vi "RDS Child Receive Message.vi"(8 "error in (no error)":errorcluster, 10 "RDS Message":refnum<class "RDS Message.lvclass">, 11 "Battery Instrument in":refnum<class "Battery Instrument.lvclass">) -> (0 "error out":errorcluster, 3 "Battery Instrument out":refnum<class "Battery Instrument.lvclass">)   [LabVIEW 2015, in "Battery Instrument.lvlib" / "Battery Instrument.lvclass"]
uses:
  Battery Instrument.lvclass
  Libraries/RDS Framework/RDS Message Class/RDS Message.lvclass
  Libraries/RDS Framework/RDS Message Class/RDS Message.lvclass/RDS Message.ctl
  Libraries/RDS Serial Handler/RDS Serial Frame.lvclass/RDS Serial Frame.ctl
  <vilib>/ActorFramework/Actor/Actor.lvclass/Actor.ctl
  <vilib>/ActorFramework/Message Enqueuer/Message Enqueuer.lvclass/Message Enqueuer.ctl
  <vilib>/ActorFramework/Message Enqueuer/Enqueue.vi
  <vilib>/ActorFramework/Message Priority Queue/Priority Enqueue.vi
  Libraries/RDS Serial Handler/RDS Serial Frame.lvclass
  <vilib>/ActorFramework/Stop Msg/Stop Msg.lvclass
  Actors/RDS Serial Instrument Actor/RDS Serial Instrument Actor.lvclass
  <vilib>/ActorFramework/Actor/Actor.lvclass
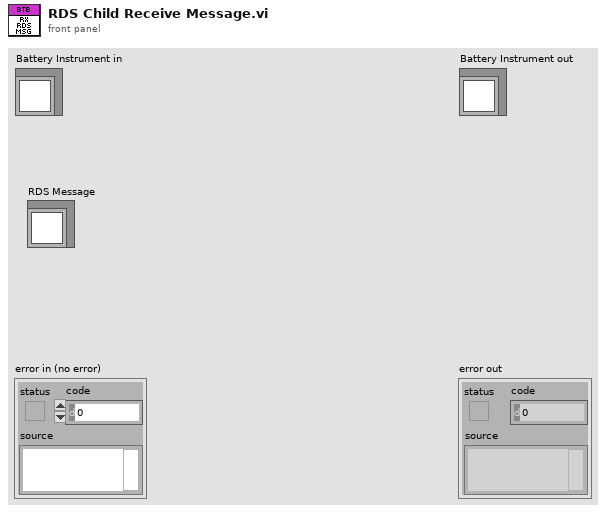
[diagram p1: front panel]
types:
  T1 = typedef "RDS Child Messages.lvlib/RDS Message ID.ctl" = enum16{"RDS Hello World", "String Message", "AIP_Status", "AIP_Command", "GPS_Data", "MCB_Command", "MCB_Status", "Compass_Data", "Depth_Data", "Battery_Data", "Contoller_State", "Set_Mag_Dev", "BTB_Shutdown", "State_Sample_Request", "State_Sample", "PID_Gains_Set", "Helm_Limiter_Set", "Helm_Heading_Command", "Helm_Steering_Command", "Helm_Status", "Controller_Message", "AIP_Set_Min_Depth", "Mission_Controller_State", "Mission_Upload", "Mission_Set_Op_and_Run", "Mission_Settings_Set"}
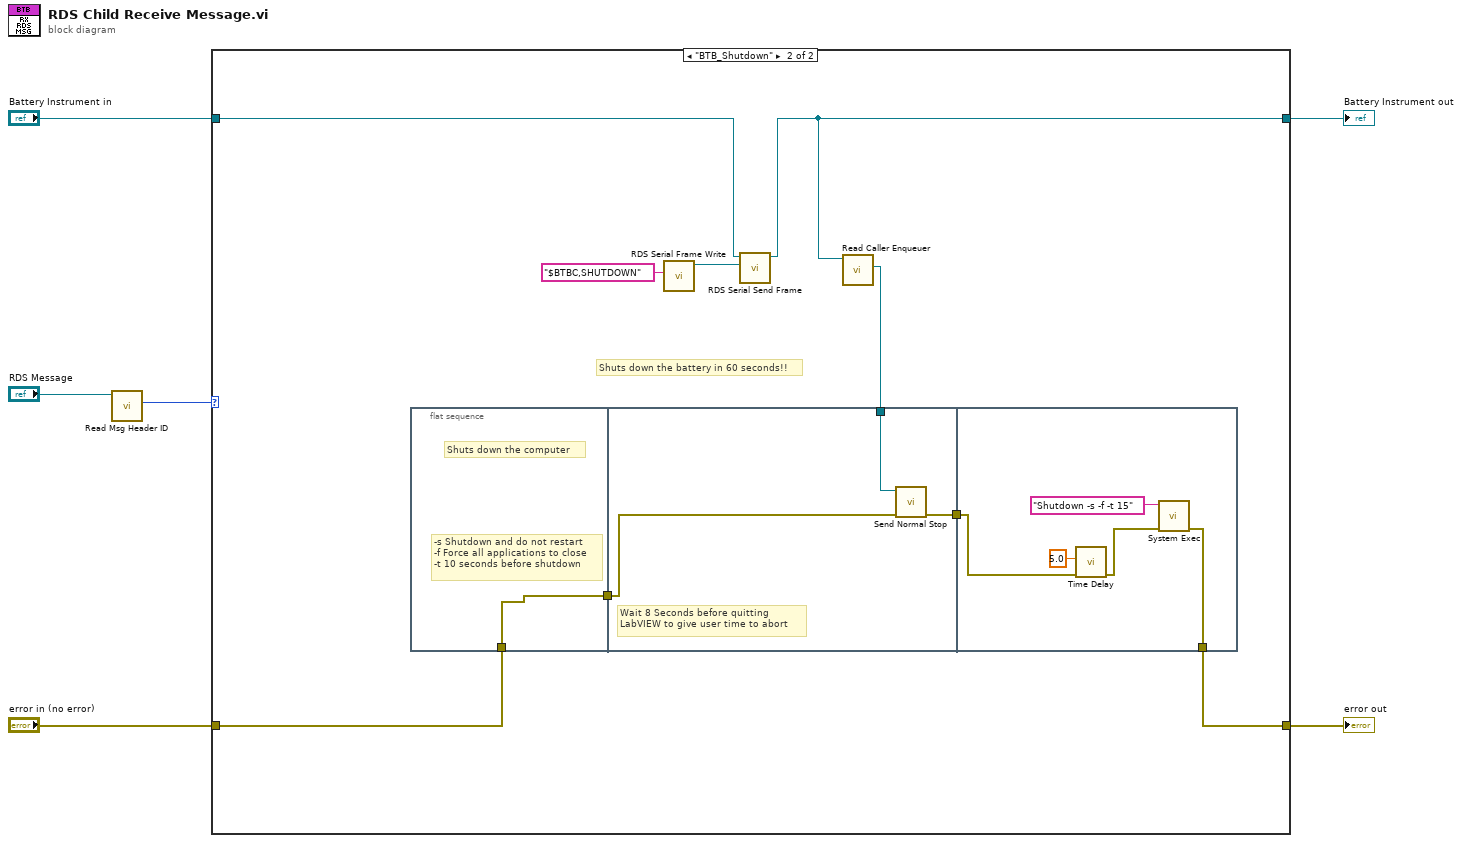
[diagram p0: block diagram]
diagram:
  n1 = call "Read Msg Header ID.vi"("RDS Message in"="RDS Message") -> ("Msg ID"=w3:T1)  [unwired: 6 in, 4 out]
  n2 = case shown="\"BTB_Shutdown\"" w3 {
    tunnel: [w7 w12] -> w6
    tunnel: "Battery Instrument in" -> [w7 w15]
    tunnel: [w8 w9] -> w2
    tunnel: "error in (no error)" -> [w8 w13]
    frame "RDS Hello World", Default {
    }
    frame "BTB_Shutdown" {
      # "Shuts down the battery in 60 seconds!!"
      n3 = flat-sequence {
        tunnel: [w18] -> w14
        tunnel: w13 -> [w18]
        tunnel: w14 -> [w19]
        tunnel: w11 -> [w21]
        tunnel: [w20] -> w10
        tunnel: w10 -> [w24]
        tunnel: [w22] -> w9
        frame #0 {
          # "-s Shutdown and do not restart\n-f Force all applications to close\n-t 10 seconds before shutdown"
          # "Shuts down the computer"
        }
        frame #1 {
          # "Wait 8 Seconds before quitting\nLabVIEW to give user time to abort"
          n4 = call <vilib>:"Send Normal Stop.vi"("error in (no error)"=w19, "Message Enqueuer"=w21) -> ("error out"=w20:errorcluster)  [unwired: 9 in]
        }
        frame #2 {
          n5 = call "Time Delay"("error in (no error)"=w24, "Delay Time (s)"=5.0) -> ("error out"=w23:errorcluster)  [unwired: 9 in]
          n6 = call <vilib>:"System Exec.vi"("error in (no error)"=w23, "command line"="Shutdown -s -f -t 15") -> ("error out"=w22:errorcluster)  [unwired: 6 in, 3 out]
        }
      }
      n7 = call "RDS Serial Frame Write.vi"("Serial String"="$BTBC,SHUTDOWN") -> ("RDS Serial Frame out"=w16:refnum<class "RDS Serial Frame.lvclass">)  [unwired: 9 in, 1 out]
      n8 = call "RDS Serial Send Frame.vi"("RDS Frame"=w16, "RDS Serial Instrument Actor in"=w15) -> ("RDS Serial Instrument Actor out"=w12:refnum<class "Battery Instrument.lvclass">)  [unwired: 8 in, 1 out]
      n9 = call <vilib>:"Read Caller Enqueuer.vi"("Actor"=w12) -> ("Caller Enqueuer"=w11:refnum<class "Message Enqueuer.lvclass">)  [unwired: 10 in]
    }
  }
  "error out" <- w2
  "Battery Instrument out" <- w6
